vi "Rio_Motion_Control_Main.vi"(8 "Error In":errorcluster) -> (0 "Error Out":errorcluster)   [LabVIEW 2017]
doc: "This VI controls the X, Y and Theta axis given posiiton and angle inputs.\n\nWritten by Stefan Clarkson, Robin Moore & Thomas Quinn 26/02/18."
uses:
  <vilib>/myRIO/Common/Instrument Driver Framework/myRIO v1.0/Encoder/typedefs/Encoder Signal Mode.ctl
  <vilib>/myRIO/Instrument Drivers/Onboard IO/Encoder/typedefs/Encoder Reference.ctl
  <vilib>/myRIO/Common/Instrument Driver Framework/Utilities/typedefs/myRIO Generic Hardware Reference.ctl
  <vilib>/myRIO/Common/Instrument Driver Framework/Utilities/typedefs/Hardware Version Enum.ctl
  <vilib>/myRIO/Common/Instrument Driver Framework/Utilities/typedefs/myRIO v1.0 Reference.ctl
  <vilib>/myRIO/Common/Instrument Driver Framework/Utilities/typedefs/Generic FPGA Reference.ctl
  <vilib>/myRIO/Common/Instrument Driver Framework/myRIO v1.0/Encoder/typedefs/Encoder Channels Enum.ctl
  <vilib>/myRIO/Common/Instrument Driver Framework/myRIO v1.0/Encoder/typedefs/Encoder Configuration v1.0.ctl
  <vilib>/userdefined/High Color/nirio_resource_hc.ctl
  <vilib>/myRIO/Common/Instrument Driver Framework/Utilities/vis/Is FPGA Ref Available.vi
  <vilib>/myRIO/Common/Instrument Driver Framework/myRIO v1.0/Encoder/vis/myRIO v1.1 Open Encoder.vi
  <vilib>/myRIO/Instrument Drivers/Onboard IO/Encoder/vis/Read.vi
  <vilib>/myRIO/Common/Instrument Driver Framework/Utilities/vis/Validate Channels.vi
  <vilib>/myRIO/Common/Instrument Driver Framework/myRIO v1.0/Encoder/vis/myRIO v1.0 Reserve Encoder.vi
  <vilib>/myRIO/Common/Instrument Driver Framework/myRIO v1.0/Encoder/vis/myRIO v1.0 Build MUX Configuration Encoder.vi
  <vilib>/myRIO/Common/Instrument Driver Framework/myRIO v1.0/Resource Manager/vis/myRIO v1.0 Reserve Channel List.vi
  <vilib>/myRIO/Common/Instrument Driver Framework/myRIO v1.0/Resource Manager/vis/myRIO v1.0 Create Configuration List.vi
  <vilib>/myRIO/Common/Instrument Driver Framework/myRIO v1.0/Resource Manager/vis/myRIO v1.0 Reserve Channel.vi
  <vilib>/myRIO/Common/Instrument Driver Framework/myRIO v1.0/Resource Manager/vis/myRIO v1.0 Unreserve Channel.vi
  <vilib>/myRIO/Common/Instrument Driver Framework/myRIO v1.0/Resource Manager/vis/myRIO v1.0 Build Mutex Name.vi
  <vilib>/Utility/VariantDataType/GetNumericInfo.vi
  <vilib>/Utility/error.llb/Error Cluster From Error Code.vi
  <vilib>/myRIO/Common/Instrument Driver Framework/myRIO v1.0/myRIO v1.1 Open.vi
  <vilib>/myRIO/Common/Instrument Driver Framework/Utilities/vis/IO Manager.vi
  <vilib>/myRIO/Common/Instrument Driver Framework/Utilities/vis/Configuration Manager.vi
  <vilib>/myRIO/Common/Instrument Driver Framework/myRIO v1.0/Resource Manager/vis/myRIO v1.0 Configure IO.vi
  <vilib>/myRIO/Common/Instrument Driver Framework/myRIO v1.0/myRIO v1.0 Close.vi
  <vilib>/myRIO/Common/Instrument Driver Framework/myRIO v1.0/Encoder/vis/myRIO v1.0 Configure Encoder.vi
  <vilib>/myRIO/Common/Instrument Driver Framework/myRIO v1.0/Encoder/vis/myRIO v1.0 Read Encoder.vi
  <vilib>/myRIO/Express VI/Onboard IO/Encoder/Encoder Express VI.xnode
  <vilib>/myRIO/Instrument Drivers/Onboard IO/Encoder/vis/myRIO Encoder Open.xnode
  <vilib>/myRIO/Common/Instrument Driver Framework/myRIO v1.0/Encoder/typedefs/Encoder Count Direction Enum.ctl
  <vilib>/myRIO/Instrument Drivers/Onboard IO/Encoder/Encoder.lvlib
panel:
  in  "Stop":bool
  in  "Theta Desired Position":dbl step=0.9
  in  "Reset X":bool
  in  "Reset Y":bool
  in  "Setpoint Y":dbl step=10000.0
  out "Y Axis":dbl[][](graph)
  out "X Axis":dbl[][](graph)
  in  "Setpoint X":dbl step=10000.0
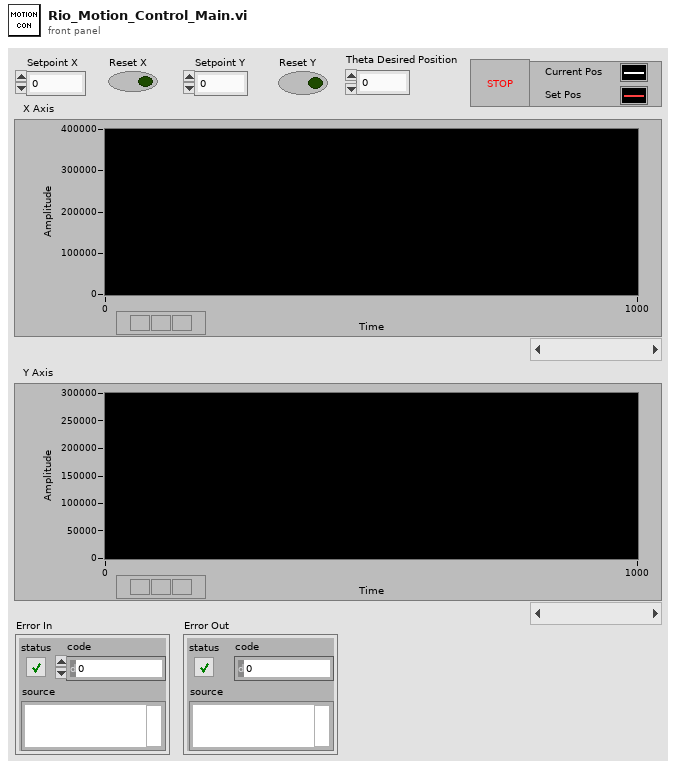
[diagram p1: front panel]
types:
  T1 = typedef "Encoder.lvlib/Encoder Reference.ctl" = cluster{"myRIO Reference":T2, "Encoder Channels Enum":T6}
  T2 = typedef "myRIO Generic Hardware Reference.ctl" = cluster{"myRIO Model":T3, "myRIO Hardware Reference":T4}
  T3 = typedef "Hardware Version Enum.ctl" = enum16{"Unknown", "myRIO-1900", "myRIO-1950", "roboRIO", "NI ELVIS RIO CM"}
  T4 = typedef "myRIO v1.0 Reference.ctl" = cluster{"Generic FPGA Reference":T5, "Allow multiple opens":bool}
  T5 = typedef "Generic FPGA Reference.ctl" = refnum<k20>
  T6 = typedef "Encoder Channels Enum.ctl" = enum16{"Not Connected", "C/ENC0", "C/ENC1", "A/ENC", "B/ENC", "DIO/ENC0", "DIO/ENC1", "DIO/ENC2", "DIO/ENC3", "DIO/ENC4"}
  T7 = typedef "Encoder Signal Mode.ctl" = enum16{"Quadrature phase signal", "Step and direction signal"}
  T8 = typedef "nirio_resource_hc.ctl" = tag
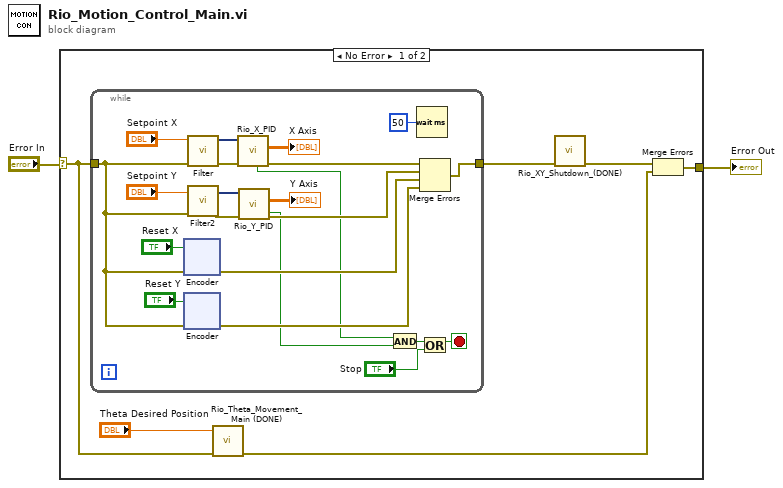
[diagram p0: block diagram]
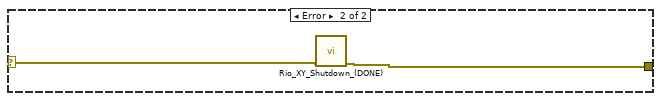
[diagram p2: hidden frame]
diagram:
  n1 = case shown="No Error" "Error In" {
    selector: "Error In" -> [w6 w123]
    tunnel: [w3 w124] -> w1
    frame No Error {
      n2 = while {
        tunnel: w6 -> [w16]
        tunnel: [w18] -> w7
        stop <- w10 stop-if-true
        n3 = xnode "Encoder"("error in (no error)"=w16, "Reset Counter"="Reset X") -> ("error out"=w15:errorcluster)  [unwired: 3 out]
        n4 = xnode "Encoder"("error in (no error)"=w16, "Reset Counter"="Reset Y") -> ("error out"=w14:errorcluster)  [unwired: 3 out]
        n5 = call "Filter"("error in (no error)"=w16, "Signal"="Setpoint X") -> ("error out"=w29:errorcluster, "Filtered Signal"=w26:dynamicdata)  [unwired: 8 in]
        n6 = call "Filter2"("error in (no error)"=w16, "Signal"="Setpoint Y") -> ("error out"=w22:errorcluster, "Filtered Signal"=w25:dynamicdata)  [unwired: 8 in]
        n7 = call "Rio_X_PID.vi"("Error In"=w29, "Setpoint"=w26) -> ("Error Out"=w19:errorcluster, "Waveform Chart"=→"X Axis":dbl[][], "Stop"=w12:bool)  [unwired: 6 in, 1 out]
        n8 = call "Rio_Y_PID.vi"("Error In"=w22, "Setpoint"=w25) -> ("Error Out"=w20:errorcluster, "Waveform Chart"=→"Y Axis":dbl[][], "Stop"=w11:bool)  [unwired: 6 in, 1 out]
        n9 = And(x=w12, y=w11) -> (x .and. y?=w13:bool)
        n10 = Wait (ms)(milliseconds to wait=u32 50) -> ()  [unwired: 1 out]
        n11 = Merge Errors(w19, w20, w15, w14) -> (w18:errorcluster)
        n12 = Or(x=w13, y="Stop") -> (x .or. y?=w10:bool)
      }
      n13 = call "Rio_Theta_Movement_Main (DONE).vi"("Desired Position"="Theta Desired Position", "Error In"=w6) -> ("error out"=w4:errorcluster)  [unwired: 9 in]
      n14 = call "Rio_XY_Shutdown_(DONE).vi"("error in (no error)"=w7) -> ("error out"=w5:errorcluster)  [unwired: 10 in]
      n15 = Merge Errors(w5, w4) -> (w3:errorcluster)
    }
    frame Error {
      n16 = call "Rio_XY_Shutdown_(DONE).vi"("error in (no error)"=w123) -> ("error out"=w124:errorcluster)  [unwired: 10 in]
    }
  }
  "Error Out" <- w1
